vi "ManualLiftControl.vi"(7 "MaxLiftIncriment":dbl, 10 "PrevLiftSetpoint":dbl, 11 "JoystickAxis":dbl[](array[numeric])) -> (2 "NewLiftSetpoint":dbl)   [LabVIEW 2014]
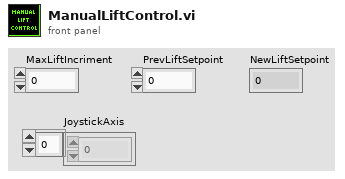
[diagram p1: front panel]
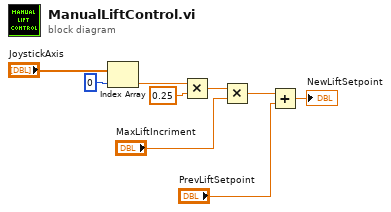
[diagram p0: block diagram]
diagram:
  n1 = Index Array(array="JoystickAxis", index=0) -> (element=w6:dbl)
  n2 = Multiply(x=w6, y=0.25) -> (x*y=w2:dbl)
  n3 = Multiply(x=w2, y="MaxLiftIncriment") -> (x*y=w5:dbl)
  n4 = Add(x=w5, y="PrevLiftSetpoint") -> (x+y=→"NewLiftSetpoint":dbl)
